vi "Status.vi"(8 "error in (no error)":errorcluster caption="错误输入（无错误）", 11 "FIFO(DBL) 输入":refnum<class "FIFO(U16).lvclass"> caption="DNL_LabVIEW Object in") -> (0 "error out":errorcluster caption="错误输出", 1 "Current Size":i32, 2 "Current Elements":u16[](array[numeric]), 3 "FIFO(DBL) 输出":refnum<class "FIFO(U16).lvclass"> caption="DNL_LabVIEW Object out")   [LabVIEW 2012, in "FIFO(U16).lvclass"]
uses:
  FIFO(U16).lvclass
  FIFO(U16).lvclass/FIFO(U16).ctl
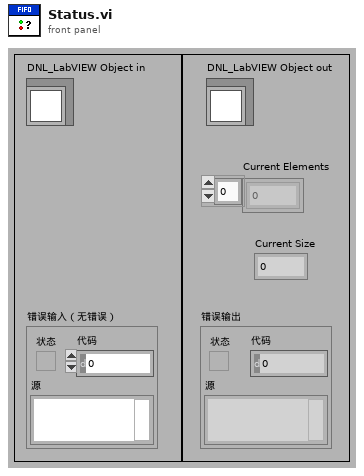
[diagram p1: front panel]
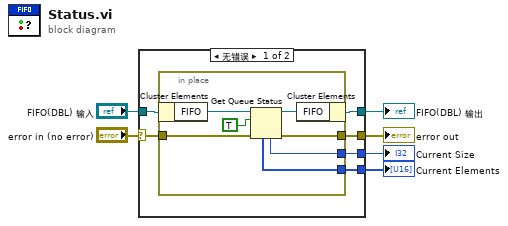
[diagram p0: block diagram]
diagram:
  n1 = case shown="无错误" "error in (no error)" {
    selector: "error in (no error)" -> [w10 w21]
    tunnel: [w9 w21] -> w5
    tunnel: [w11 w20] -> w3
    tunnel: "FIFO(DBL) 输入" -> [w12 w20]
    tunnel: [w8 _] -> w2
    tunnel: [w7 _] -> w1
    frame No Error {
      n2 = in-place {
        in-place-border: w10 -> [w17]
        in-place-border: [w16] -> w9
        in-place-border: [w14] -> w8
        in-place-border: [w13] -> w7
        n3 = in-place-cluster #1(w12) -> ("FIFO"=w19:refnum<queue>)
        n4 = Get Queue Status(queue=w19, return elements? (F)=TRUE ("返回元素？(F)"), error in (no error)=w17) -> (queue out=w18:refnum<queue>, error out=w16:errorcluster, # elements in queue=w14:i32, elements=w13:u16[])  [unwired: 4 out]
        n5 = in-place-cluster #1("FIFO"=w18) -> (w11:refnum<class "FIFO(U16).lvclass">)
      }
    }
    frame Error {
    }
  }
  "error out" <- w5
  "FIFO(DBL) 输出" <- w3
  "Current Elements" <- w1
  "Current Size" <- w2
